vi "Jeffress_model_v005.vi"() -> ()   [LabVIEW 2019]
panel:
  out "Index":string
  out "new picture":picture
  in  "stop":bool
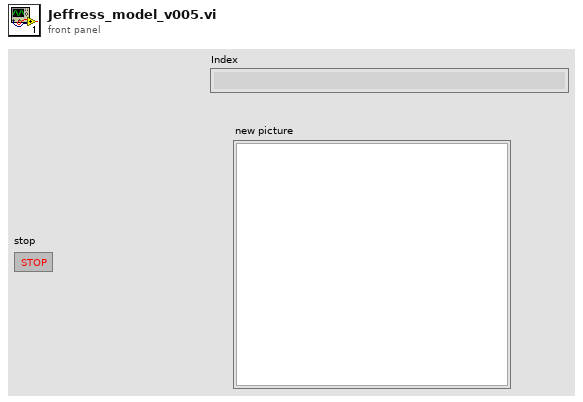
[diagram p1: front panel]
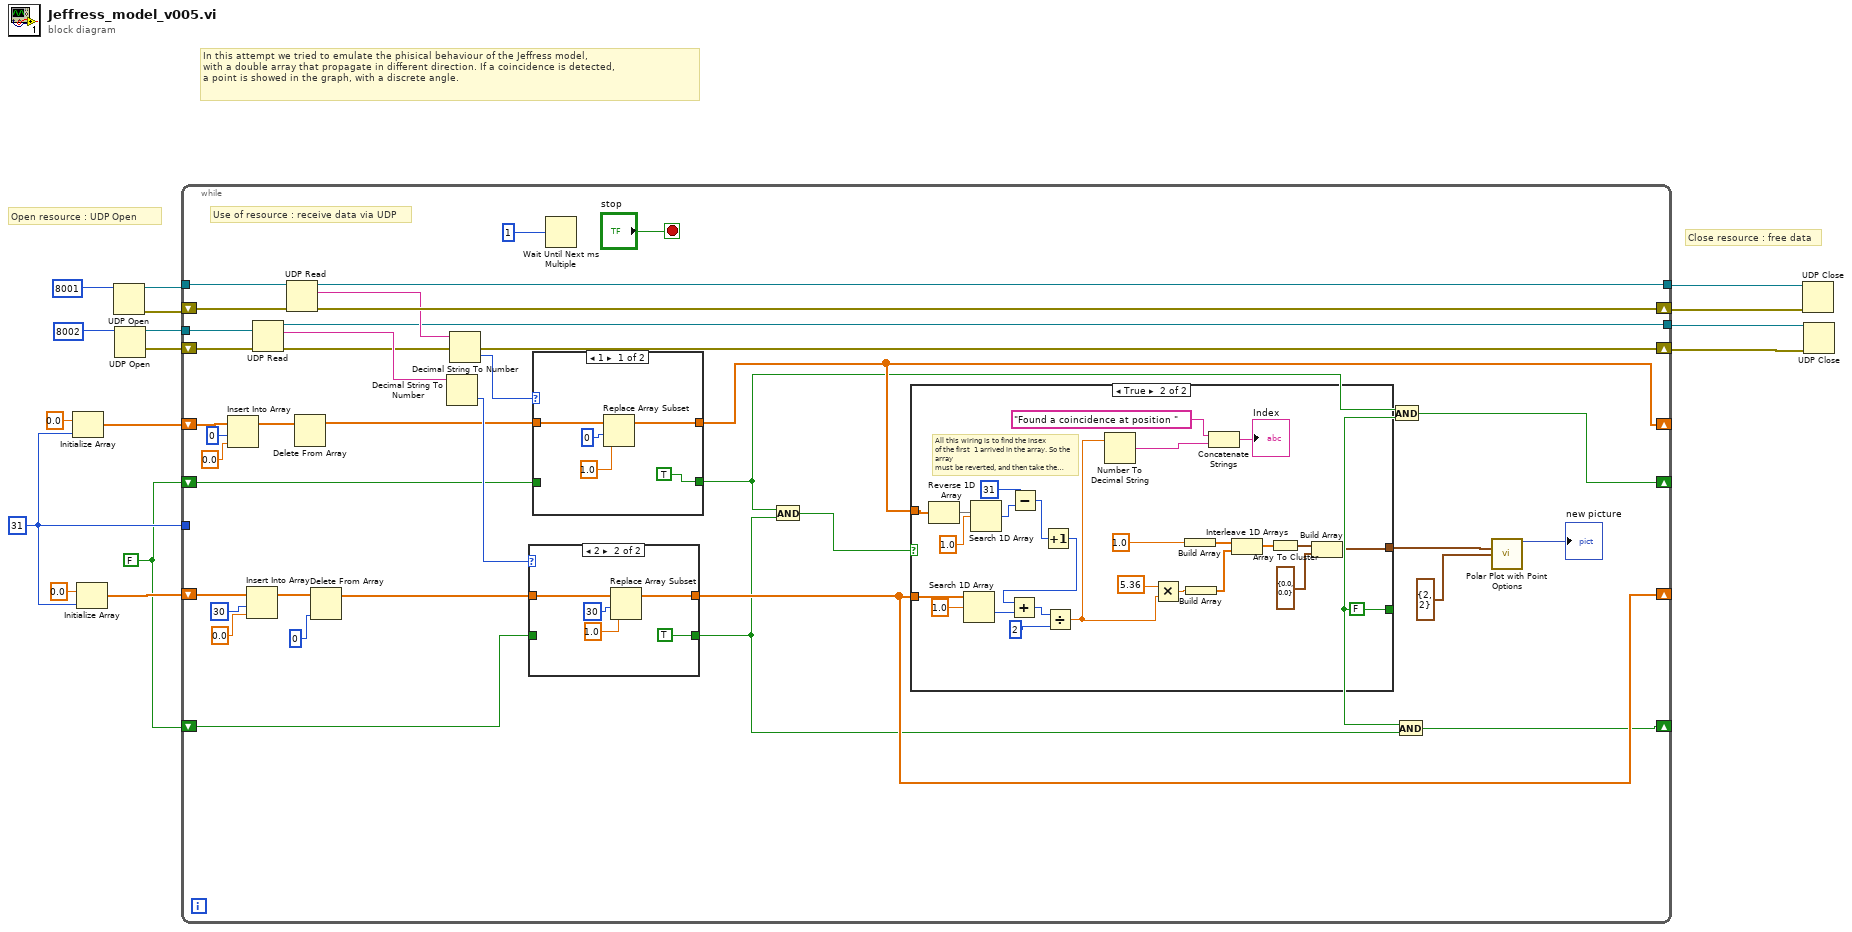
[diagram p0: block diagram]
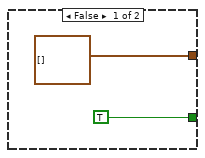
[diagram p2: hidden frame]
diagram:
  w1 = FALSE
  w2 = 31 ("dimension size")
  # "In this attempt we tried to emulate the phisical behaviour of the Jeffress model,\nwith a double array that propagate in different direction. If a coincidence is detected,\na point is showed in the graph, with a discrete angle."
  # "Close resource : free data"
  # "Open resource : UDP Open"
  n1 = Initialize Array(0.0 ("element"), w2) -> (w5:dbl[])
  n2 = Initialize Array(0.0 ("element"), w2) -> (w3:dbl[])
  n3 = UDP Open(11:u16 8001) -> (port=w14:refnum<k16>, 0:w16:errorcluster)  [unwired: 4 in, 1 out]
  n4 = UDP Open(11:u16 8002) -> (port=w10:refnum<k16>, 0:w9:errorcluster)  [unwired: 4 in, 1 out]
  n5 = while {
    tunnel: w14 -> [w50]
    tunnel: [w49] -> w13
    shift-right: [w52] -> w15
    shift-left: w16 -> [w51]
    tunnel: w10 -> [w43]
    shift-right: [w39] -> w8
    shift-left: w9 -> [w42]
    tunnel: [w40] -> w7
    shift-right: [w26] -> _
    shift-left: w5 -> [w38]
    shift-right: [w25] -> _
    shift-left: w3 -> [w30]
    tunnel: w2 -> [_]
    shift-right: [w19] -> _
    shift-left: w1 -> [w24]
    shift-right: [w18] -> _
    shift-left: w1 -> [w23]
    stop <- "stop" stop-if-true
    # "Use of resource : receive data via UDP"
    n6 = Insert Into Array(array=w38, index=0, new element=0.0 ("new element/subarray")) -> (w35:dbl[])
    n7 = Insert Into Array(array=w30, index=30, new element=0.0 ("new element/subarray")) -> (w31:dbl[])
    n8 = UDP Read(connection ID=w43, 8:w42) -> (data out=w44:string, error out=w39:errorcluster, 3:w40:refnum<k16>)  [unwired: 2 in, 2 out]
    n9 = UDP Read(connection ID=w50, 8:w51) -> (data out=w45:string, error out=w52:errorcluster, 3:w49:refnum<k16>)  [unwired: 2 in, 2 out]
    n10 = Delete From Array(array=w35) -> (array with subset deleted=w34:dbl[])  [unwired: 2 in, 1 out]
    n11 = Delete From Array(array=w31, index=0) -> (array with subset deleted=w28:dbl[])  [unwired: 1 in, 1 out]
    n12 = Decimal String To Number(string=w44) -> (number=w41:i32)  [unwired: 2 in, 1 out]
    n13 = Decimal String To Number(string=w45) -> (number=w46:i32)  [unwired: 2 in, 1 out]
    n14 = case shown="2" w41 {
      tunnel: [w84 w87] -> w25
      tunnel: w28 -> [w84 w86]
      tunnel: [w83 TRUE] -> w22
      tunnel: w23 -> [w83 _]
      frame Default {
      }
      frame 2 {
        n15 = Replace Array Subset(array=w86, new element=1.0 ("new element/subarray"), index=30) -> (w87:dbl[])
      }
    }
    n16 = case shown="1" w46 {
      tunnel: [w92 w96] -> w26
      tunnel: w34 -> [w91 w96]
      tunnel: [TRUE w95] -> w20
      tunnel: w24 -> [_ w95]
      frame 1 {
        n17 = Replace Array Subset(array=w91, new element=1.0 ("new element/subarray"), index=0) -> (w92:dbl[])
      }
      frame Default {
      }
    }
    n18 = Wait Until Next ms Multiple(millisecond multiple=u32 1) -> ()  [unwired: 1 out]
    n19 = And(x=w20, y=w22) -> (x .and. y?=w27:bool)
    n20 = case shown="True" w27 {
      tunnel: [cluster{"magnitude":dbl, "phase":dbl}[] [] ("data array [mag, phase (deg)]") w58] -> w17
      tunnel: w26 -> [_ w71]
      tunnel: w25 -> [_ w78]
      tunnel: [TRUE FALSE] -> w21
      frame False {
      }
      frame True {
        # "All this wiring is to find the insex\nof the first  1 arrived in the array. So the array \nmust be reverted, and then take the original \nindex."
        n21 = Reverse 1D Array(array=w71) -> (reversed array=w70:dbl[])
        n22 = Search 1D Array(1D array=w78, element=1.0) -> (index of element=w76:i32)  [unwired: 1 in]
        n23 = Search 1D Array(1D array=w70, element=1.0) -> (index of element=w66:i32)  [unwired: 1 in]
        n24 = Subtract(x=31, y=w66) -> (x-y=w64:i32)
        n25 = Increment(x=w64) -> (x+1=w63:i32)
        n26 = Add(x=w63, y=w76) -> (x+y=w75:i32)
        n27 = Divide(x=w75, y=2) -> (x/y=w72:dbl)
        n28 = Number To Decimal String(number=w72) -> (decimal integer string=w81:string)  [unwired: 1 in]
        n29 = Multiply(x=5.36, y=w72) -> (x*y=w82:dbl)
        n30 = Build Array(1.0) -> (w62:dbl[])
        n31 = Build Array(w82) -> (w61:dbl[])
        n32 = Concatenate Strings("Found a coincidence at position ", w81) -> (→"Index":string)
        n33 = Interleave 1D Arrays(w62, w61) -> (w60:dbl[])
        n34 = Array To Cluster(array=w60) -> (cluster=w59:cluster{"[0]":dbl, "[1]":dbl})
        n35 = Build Array(w59, cluster{"[0]":dbl, "[1]":dbl} {"[0]"=0.0, "[1]"=0.0} ("element")) -> (w58:cluster{"[0]":dbl, "[1]":dbl}[])
      }
    }
    n36 = And(x=w20, y=w21) -> (x .and. y?=w19:bool)
    n37 = And(x=w21, y=w22) -> (x .and. y?=w18:bool)
    n38 = call <vilib>:"Polar Plot with Point Options.vi"("data array [mag, phase (deg)]"=w17, "top left point(0, 0)"=cluster{"x":i16, "y":i16} {"x"=2, "y"=2}) -> ("new picture"=→"new picture":picture)  [unwired: 13 in]
  }
  n39 = UDP Close(connection ID=w13, 8:w15) -> ()  [unwired: 2 out]
  n40 = UDP Close(connection ID=w7, 8:w8) -> ()  [unwired: 2 out]
